vi "HART.vi"(4 "Error In":errorcluster, 7 "Command":string) -> (0 "Error Out":errorcluster, 3 "Response":string)   [LabVIEW 2018]
uses:
  MOKO_LabViewLibrary/MokoLowLevel/MokoLowLovelControl/MLLC_ConnectCluster.ctl
  MOKO_LabViewLibrary/MokoLowLevel/MokoLowLovelControl/MLLC_InterfaceType.ctl
  MOKO_LabViewLibrary/MokoLowLevel/MokoLowLovelControl/MLLC_OpenedSession.ctl
  MOKO_LabViewLibrary/MokoLowLevel/MokoLowLovelControl/MLLC_InterfaceSettings.ctl
  MOKO_LabViewLibrary/MokoLowLevel/MokoLowLovelControl/MLLC_InterfaceKind.ctl
panel:
  in  "Settings":T6={"Saved Data"=variant, "Data"={"Connect"={"InterfaceType"=enum."VISA", "OpenedSession"="", "InterfaceSettings"={"Interface"=enum."RS232", "EOS 4 read"=enum."LF (\\n)", "EOS 4 write"=enum."LF (\\n)", "TMO, ms"=10000, "Sett"=variant(cluster{"Baud Rate":u32, "Data Bits":u16, "Parity":u16, "Stop Bits":u16, "Flow Control":u16, "Eho":bool} {"Baud Rate"=75, "Data Bits"=0, "Parity"=0, "Stop Bits"=0, "Flow Control"=0, "Eho"=FALSE})}}, "Value"={"I"=0.0, "P"=0.0, "T"=0.0}, "String"="empty"}}
  in  "Error Code":u32
  in  "Driver Name":string="HART"
  in  "Mode":T7(ring)=enum."Check"
  # "HART"
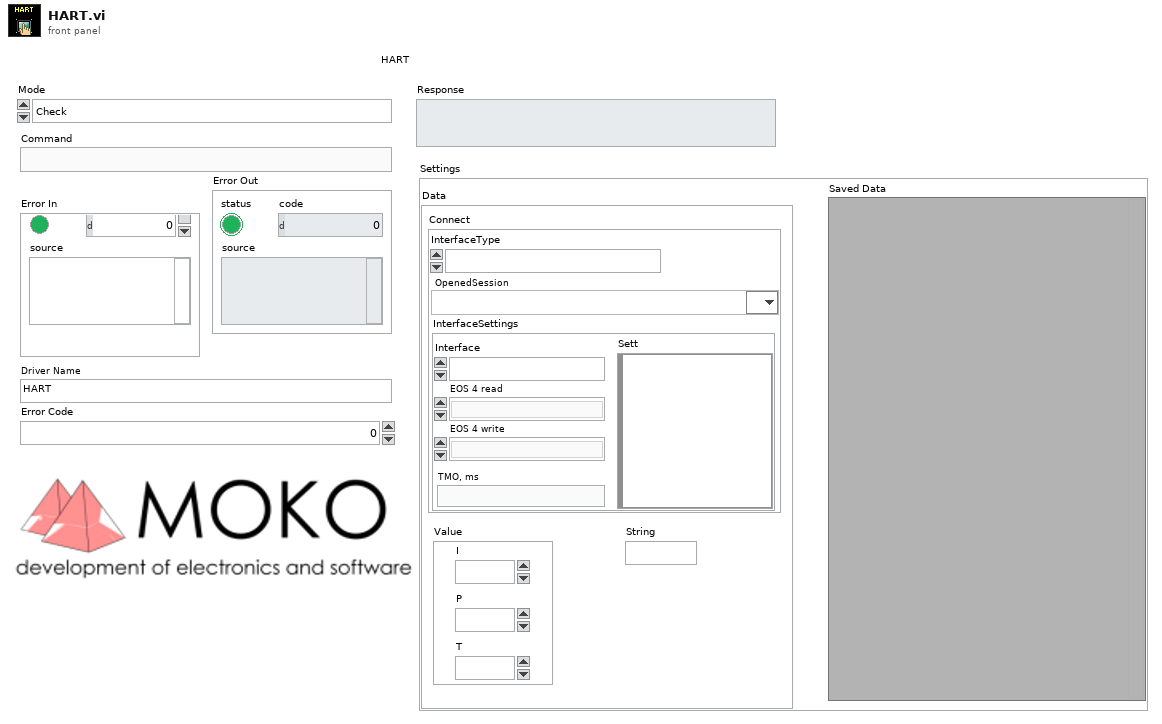
[diagram p1: front panel]
types:
  T1 = typedef "MLLC_ConnectCluster.ctl" = cluster{"InterfaceType":T2, "OpenedSession":T3, "InterfaceSettings":T4}
  T2 = typedef "MLLC_InterfaceType.ctl" = enum16{"VISA", "Prologix USB-GPIB"}
  T3 = typedef "MLLC_OpenedSession.ctl" = refnum<visa-resource-name>
  T4 = typedef "MLLC_InterfaceSettings.ctl" = cluster{"Interface":T5, "EOS 4 read":enum16{"Default (=EOS 4 write)", "CR (\\r)", "LF (\\n)", "None"}, "EOS 4 write":enum16{"CR+LF (\\r\\n)", "CR (\\r)", "LF (\\n)", "None"}, "TMO, ms":i32, "Sett":variant}
  T5 = typedef "MLLC_InterfaceKind.ctl" = enum16{"RS232", "GPIB", "USB", "Ethernet", "another"}
  T6 = cluster{"Saved Data":variant, "Data":cluster{"Connect":T1, "Value":cluster{"I":dbl, "P":dbl, "T":dbl}, "String":string}}
  T7 = enum16{"get", "set", "close", "Init", "Check", "ID"}
  T8 = cluster{"Connect":T1, "Value":cluster{"I":dbl, "P":dbl, "T":dbl}, "String":string}
  T9 = typedef "MLLC_Mode.ctl" = enum16{"get", "set", "close", "Init", "Check"}
  T10 = typedef "MLLC_Error.ctl" = errorcluster
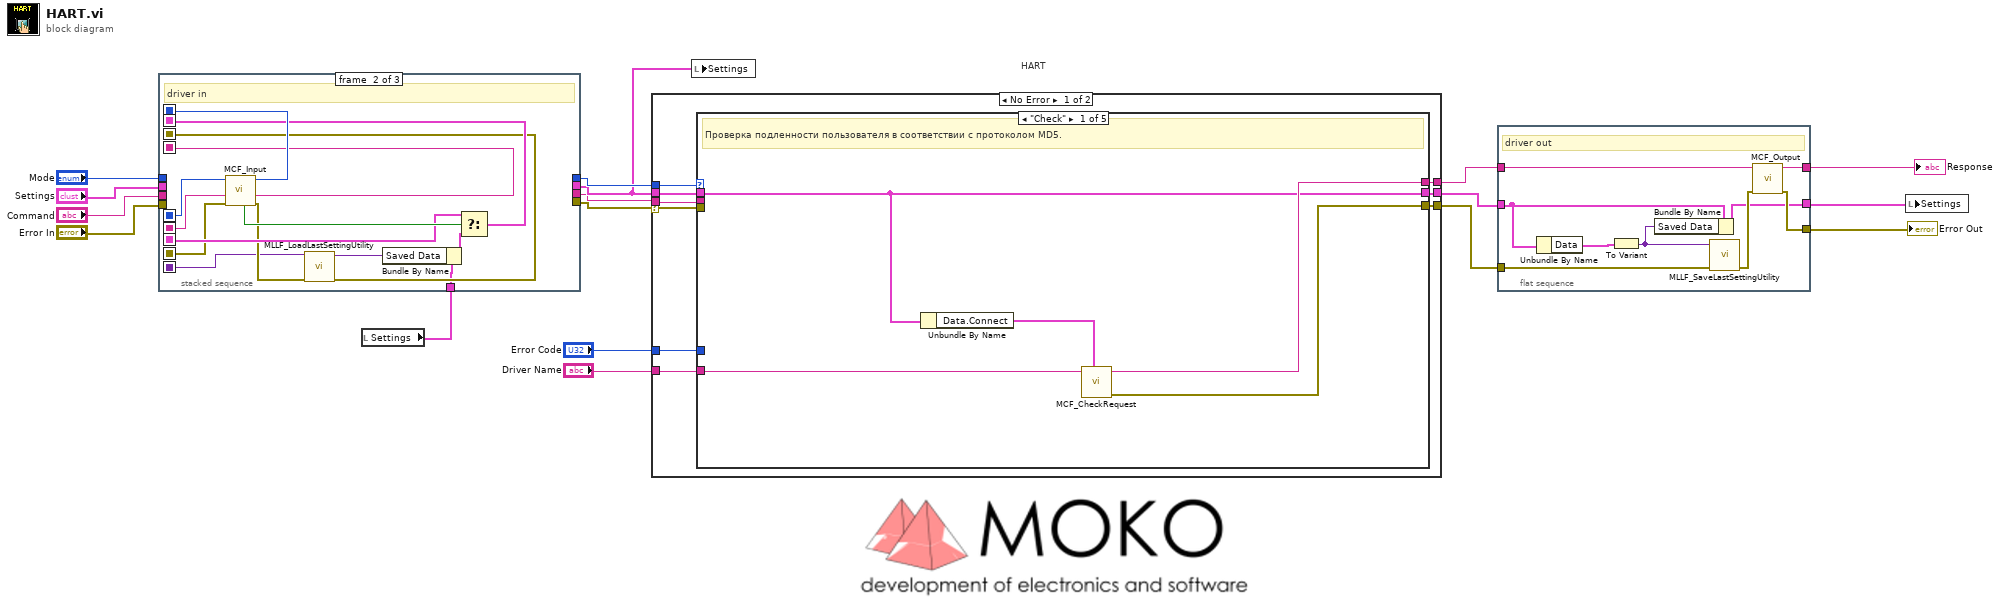
[diagram p0: block diagram]
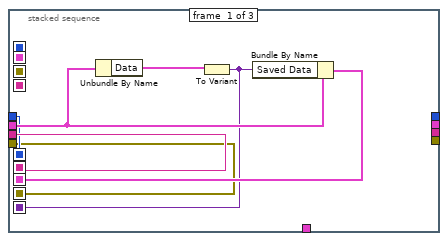
[diagram p2: hidden frame]
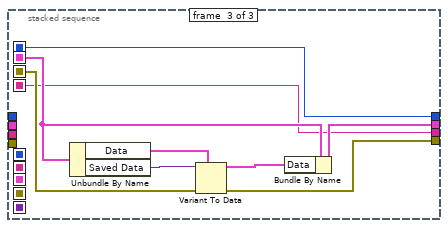
[diagram p3: hidden frame]
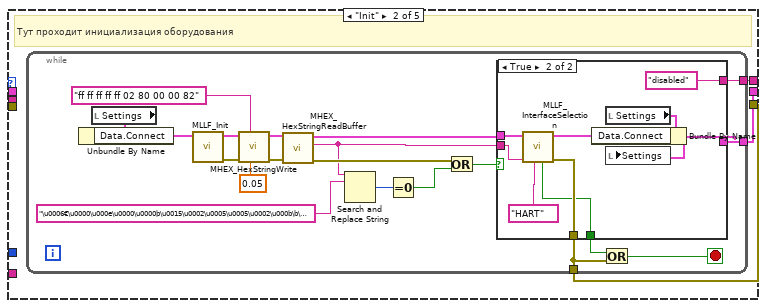
[diagram p4: hidden frame]
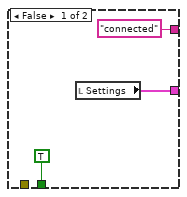
[diagram p5: hidden frame]
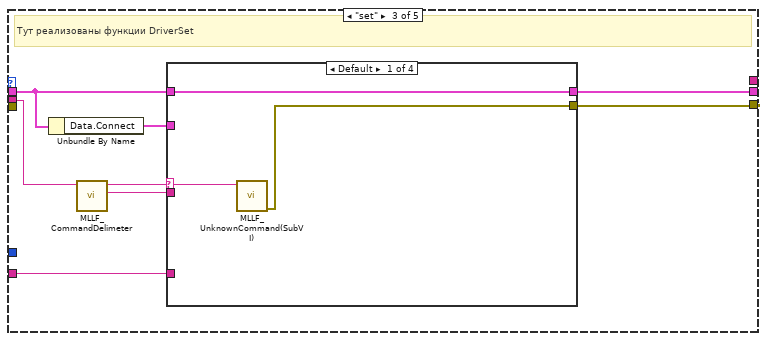
[diagram p6: hidden frame]
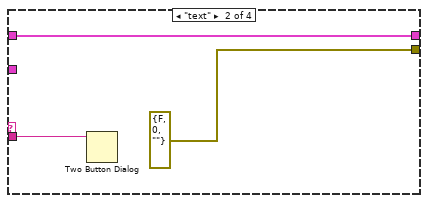
[diagram p7: hidden frame]
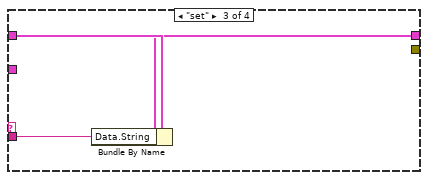
[diagram p8: hidden frame]
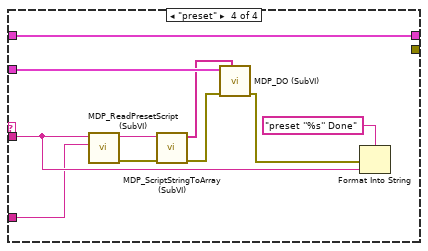
[diagram p9: hidden frame]
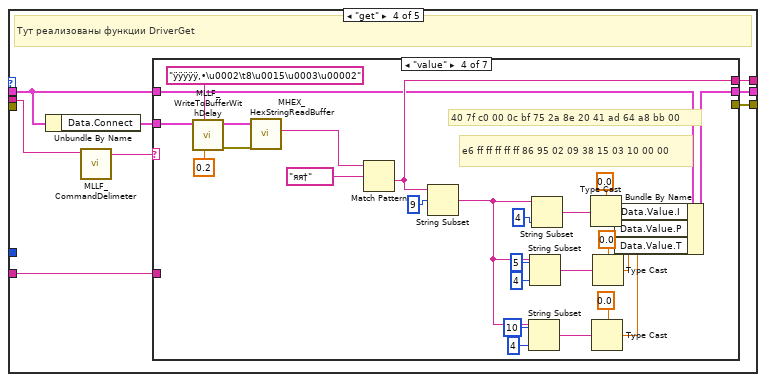
[diagram p10: hidden frame]
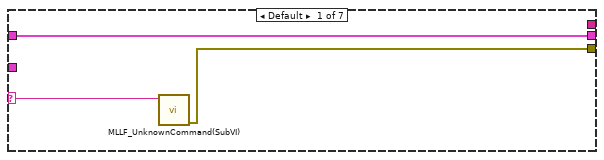
[diagram p11: hidden frame]
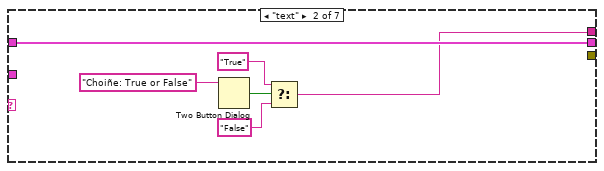
[diagram p12: hidden frame]
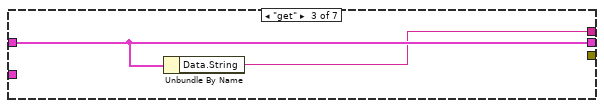
[diagram p13: hidden frame]
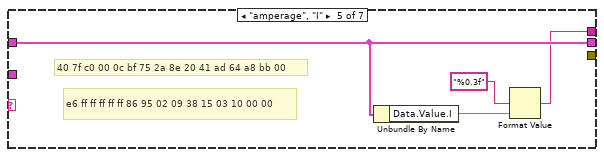
[diagram p14: hidden frame]
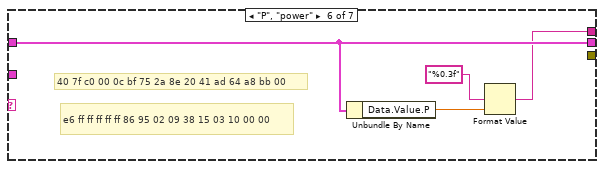
[diagram p15: hidden frame]
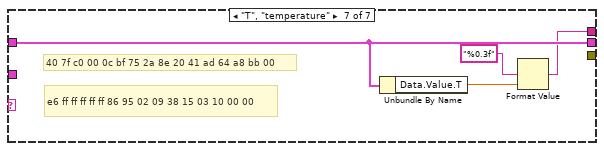
[diagram p16: hidden frame]
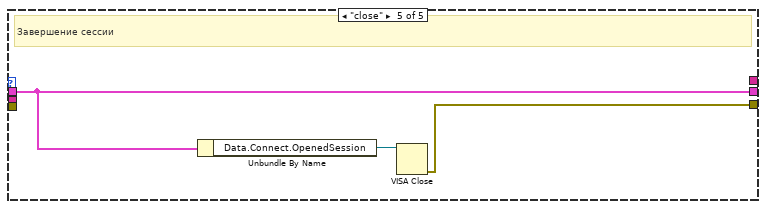
[diagram p17: hidden frame]
diagram:
  # "HART"
  n1 = local read "Settings"() -> (w13:T6)
  n2 = stacked-sequence {
    seq-local: [w20 _ _] -> [_ w36 _]
    seq-local: [w19 _ _] -> [_ w37 _]
    seq-local: [w22 _ _] -> [_ w32 _]
    seq-local: [w18 _ _] -> [_ w31 _]
    seq-local: [w21 _ _] -> [_ w27 _]
    seq-local: [_ w28 _] -> [_ _ w44]
    seq-local: [_ w38 _] -> [_ _ w41]
    seq-local: [_ w35 _] -> [_ _ w40]
    seq-local: [_ w34 _] -> [_ _ w45]
    tunnel: "Command" -> [w20 _ _]
    tunnel: "Mode" -> [w19 _ _]
    tunnel: "Error In" -> [w18 _ _]
    tunnel: "Settings" -> [w23 _ _]
    tunnel: w13 -> [_ w26 _]
    tunnel: [_ _ w40] -> w12
    tunnel: [_ _ w43] -> w14
    tunnel: [_ _ w42] -> w11
    tunnel: [_ _ w41] -> w15
    frame #0 {
      n3 = Unbundle By Name(w23) -> ("Data"=w24:T8)
      n4 = To Variant(anything=w24) -> (Variant=w21:variant)
      n5 = Bundle By Name(cluster=w23, "Saved Data"=w21) -> (w22:T6)
    }
    frame #1 {
      # "driver in"
      n6 = call "MCF_Input.vi"("Error In"=w31, "Command in"=w36, "Mode in"=w37) -> ("Error Out"=w30:errorcluster, "Command out"=w35:string, "Mode out"=w38:T9, "Boolean"=w33:bool)  [unwired: 5 in]
      n7 = call "MLLF_LoadLastSettingUtility.vi"("Error In"=w30, "Save data in"=w27) -> ("Error Out"=w28:errorcluster, "Save data out"=w25:variant)  [unwired: 8 in]
      n8 = Bundle By Name(cluster=w26, "Saved Data"=w25) -> (w29:T6)
      n9 = Select(t=w32, s=w33, f=w29) -> (s? t:f=w34:T6)
    }
    frame #2 {
      n10 = Unbundle By Name(w45) -> ("Data"=w46:T8, "Saved Data"=w39:variant)
      n11 = Variant To Data(error in=w44, type=w46, Variant=w39) -> (data=w47:T8, error out=w42:errorcluster)
      n12 = Bundle By Name(cluster=w45, "Data"=w47) -> (w43:T6)
    }
  }
  n13 = case shown="No Error" w11 {
    selector: w11 -> [w53 w185]
    tunnel: [w48 w185] -> w4
    tunnel: w15 -> [w56 _]
    tunnel: [w55 _] -> w6
    tunnel: w12 -> [w54 _]
    tunnel: w14 -> [w50 w184]
    tunnel: "Error Code" -> [w52 _]
    tunnel: "Driver Name" -> [w51 _]
    tunnel: [w49 w184] -> w5
    frame No Error {
      n14 = case shown="\"Check\"" w56 {
        tunnel: [w60 w63 _ w125 _] -> w55
        tunnel: w54 -> [_ _ w100 w128 _]
        tunnel: w53 -> [_ _ _ _ _]
        tunnel: w52 -> [_ _ _ _ _]
        tunnel: w51 -> [w61 _ w102 w126 _]
        tunnel: w50 -> [w58 _ w104 w131 w182]
        tunnel: [w58 w64 w103 w130 w182] -> w49
        tunnel: [w59 w62 w97 w124 w181] -> w48
        frame "Check" {
          # "Проверка подленности пользователя в соответствии с протоколом MD5."
          n15 = Unbundle By Name(w58) -> ("Data.Connect"=w57:T1)
          n16 = call "MCF_CheckRequest.vi"("Permanent data.Connect"=w57, "Driver Name"=w61) -> ("Error Out"=w59:errorcluster, "Output String"=w60:string)  [unwired: 8 in]
        }
        frame "Init" {
          # "Тут проходит инициализация оборудования"
          n17 = while {
            tunnel: [w81] -> w64
            tunnel: [w79] -> w63
            tunnel: [w66] -> w62
            stop <- w83 stop-if-true
            n18 = local read "Settings"() -> (w82:T6)
            n19 = Unbundle By Name(w82) -> ("Data.Connect"=w80:T1)
            n20 = call "MLLF_Init.vi"("DriverConnect in"=w80) -> ("Error Out"=w76:errorcluster, "DriverConnect out"=w77:T1)  [unwired: 7 in]
            n21 = call "MHEX_HexStringWrite.vi"("Delay Time (s)"=0.05, "Command"="ff ff ff ff ff 02 80 00 00 82" ("commands"), "error in"=w76, "DriverConnect in"=w77) -> ("error out"=w74:T10, "DriverConnect out"=w75:T1)  [unwired: 6 in]
            n22 = call "MHEX_HexStringReadBuffer.vi"("error in"=w74, "DriverConnect in"=w75) -> ("error out"=w69:T10, "String from device out"=w65:string, "DriverConnect out"=w73:T1)  [unwired: 6 in, 1 out]
            n23 = Search and Replace String(input string=w65, search string="\u0006€\u0000\u000e\u0000\u0000þ\u0015\u0002\u0005\u0005\u0002\u000b\b\u0000\t8\u0015D\u0000") -> (number of replacements=w71:i32)  [unwired: 6 in, 3 out]
            n24 = Equal To 0?(x=w71) -> (x = 0?=w70:bool)
            n25 = Or(x=w69, y=w70) -> (x .or. y?=w68:bool)
            n26 = case shown="True" w68 {
              tunnel: w73 -> [_ w95]
              tunnel: [TRUE w90] -> w84
              tunnel: [_ w96] -> w66
              tunnel: [w86 w91] -> w81
              tunnel: ["connected" "disabled"] -> w79
              tunnel: w65 -> [_ w88]
              frame False {
                n27 = local read "Settings"() -> (w86:T6)
              }
              frame True {
                n28 = call "MLLF_InterfaceSelection.vi"("Driver Name"="HART" ("String"), "Answer:"=w88, "DriverConnect in"=w95) -> ("error out"=w96:T10, "DriverConnect out"=w93:T1, "stop init?"=w90:bool)  [unwired: 4 in, 2 out]
                n29 = local read "Settings"() -> (w92:T6)
                n30 = Bundle By Name(cluster=w92, "Data.Connect"=w93) -> (w91:T6)
                n31 = local write "Settings"(w91) -> ()
              }
            }
            n32 = Or(x=w84, y=w66) -> (x .or. y?=w83:bool)
          }
        }
        frame "set" {
          # "Тут реализованы функции DriverSet"
          n33 = Unbundle By Name(w104) -> ("Data.Connect"=w101:T1)
          n34 = call "MLLF_CommandDelimeter.vi"("command with param"=w100) -> ("param 1"=w98:string, "command"=w99:string)  [unwired: 6 in, 3 out]
          n35 = case shown="Default" w99 {
            selector: w99 -> [w106 _ _ _]
            tunnel: [w107 w110 w112 w114] -> w103
            tunnel: w104 -> [w107 w110 w113 w114]
            tunnel: w101 -> [_ _ _ w118]
            tunnel: w98 -> [_ w108 w111 w117]
            tunnel: [w105 errorcluster {"status"=FALSE, "code"=0, "source"=""} ("error IO") _ _] -> w97
            tunnel: w102 -> [_ _ _ w116]
            frame Default {
              n36 = call "MLLF_UnknownCommand(SubVI).vi"("Unknown command"=w106) -> ("error out"=w105:errorcluster)  [unwired: 10 in]
            }
            frame "text" {
              n37 = Two Button Dialog(message=w108) -> ()  [unwired: 2 in, 1 out]
            }
            frame "set" {
              n38 = Bundle By Name(cluster=w113, "Data.String"=w111) -> (w112:T6)
            }
            frame "preset" {
              n39 = call "MDP_ReadPresetScript (SubVI).vi"("Driver Name"=w116, "String in"=w117) -> ("Error Out"=w121:errorcluster, "String out"=w122:string)  [unwired: 8 in]
              n40 = call "MDP_ScriptStringToArray (SubVI).vi"("Error In"=w121, "String script"=w122) -> ("Error Out"=w123:errorcluster, "Array script"=w115:string[])  [unwired: 8 in]
              n41 = call "MDP_DO (SubVI).vi"("Array script"=w115, "Error in (no error)"=w123, "DriverConnect in"=w118) -> ("Error Out"=w119:errorcluster)  [unwired: 7 in, 1 out]
              n42 = Format Into String(format string="preset ''%s'' Done" ("Befor substring"), error in=w119, w117) -> ()  [unwired: 1 in, 2 out]
            }
          }
        }
        frame "get" {
          # "Тут реализованы функции DriverGet"
          n43 = Unbundle By Name(w131) -> ("Data.Connect"=w129:T1)
          n44 = call "MLLF_CommandDelimeter.vi"("command with param"=w128) -> ("command"=w127:string)  [unwired: 6 in, 4 out]
          n45 = case shown="\"value\"" w127 {
            selector: w127 -> [w133 _ _ _ _ _ _]
            tunnel: w129 -> [_ _ _ w167 _ _ _]
            tunnel: w131 -> [w134 w140 w142 w148 w172 w176 w180]
            tunnel: [w134 w140 w142 w144 w172 w176 w180] -> w130
            tunnel: [_ w135 w141 w162 w169 w173 w177] -> w125
            tunnel: [w132 _ _ _ _ _ _] -> w124
            tunnel: w126 -> [_ _ _ _ _ _ _]
            frame Default {
              n46 = call "MLLF_UnknownCommand(SubVI).vi"("Unknown command"=w133) -> ("error out"=w132:errorcluster)  [unwired: 10 in]
            }
            frame "text" {
              n47 = Two Button Dialog(message="Choiñe: True or False") -> (T button?=w139:bool)  [unwired: 2 in]
              n48 = Select(t="True" ("string"), s=w139, f="False" ("string")) -> (s? t:f=w135:string)
            }
            frame "get" {
              n49 = Unbundle By Name(w142) -> ("Data.String"=w141:string)
            }
            frame "value" {
              # "40 7f c0 00 0c bf 75 2a 8e 20 41 ad 64 a8 bb 00"
              # "e6 ff ff ff ff ff 86 95 02 09 38 15 03 10 00 00"
              n50 = call "MLLF_WriteToBufferWithDelay.vi"("Delay Time ( 0,05 s)"=0.2 ("Delay Time (s)"), "Command"="ÿÿÿÿÿ‚•\u0002\t8\u0015\u0003\u00002", "DriverConnect in"=w167) -> ("Error Out"=w165:errorcluster, "DriverConnect out"=w166:T1)  [unwired: 7 in]
              n51 = call "MHEX_HexStringReadBuffer.vi"("error in"=w165, "DriverConnect in"=w166) -> ("String from device out"=w143:string)  [unwired: 6 in, 3 out]
              n52 = Match Pattern(string=w143, regular expression="яя†" ("HEX Response")) -> (after substring=w162:string)  [unwired: 1 in, 3 out]
              n53 = String Subset(string=w162, offset (0)=9) -> (substring=w150:string)  [unwired: 1 in]
              n54 = String Subset(string=w150, offset (0)=10, length (rest)=4 ("offset (0)")) -> (substring=w149:string)
              n55 = String Subset(string=w150, offset (0)=5, length (rest)=4 ("offset (0)")) -> (substring=w155:string)
              n56 = String Subset(string=w150, length (rest)=4 ("offset (0)")) -> (substring=w158:string)  [unwired: 1 in]
              n57 = Type Cast(type=sgl 0.0, x=w158) -> (*(type *) &x=w147:sgl)
              n58 = Type Cast(type=sgl 0.0, x=w149) -> (*(type *) &x=w145:sgl)
              n59 = Type Cast(type=sgl 0.0, x=w155) -> (*(type *) &x=w146:sgl)
              n60 = Bundle By Name(cluster=w148, "Data.Value.I"=w147, "Data.Value.P"=w146, "Data.Value.T"=w145) -> (w144:T6)
            }
            frame "amperage", "I" {
              # "40 7f c0 00 0c bf 75 2a 8e 20 41 ad 64 a8 bb 00"
              # "e6 ff ff ff ff ff 86 95 02 09 38 15 03 10 00 00"
              n61 = Unbundle By Name(w172) -> ("Data.Value.I"=w171:dbl)
              n62 = Format Value(format string="%0.3f", value (0)=w171) -> (output string=w169:string)  [unwired: 1 in]
            }
            frame "P", "power" {
              # "40 7f c0 00 0c bf 75 2a 8e 20 41 ad 64 a8 bb 00"
              # "e6 ff ff ff ff ff 86 95 02 09 38 15 03 10 00 00"
              n63 = Unbundle By Name(w176) -> ("Data.Value.P"=w175:dbl)
              n64 = Format Value(format string="%0.3f", value (0)=w175) -> (output string=w173:string)  [unwired: 1 in]
            }
            frame "T", "temperature" {
              # "40 7f c0 00 0c bf 75 2a 8e 20 41 ad 64 a8 bb 00"
              # "e6 ff ff ff ff ff 86 95 02 09 38 15 03 10 00 00"
              n65 = Unbundle By Name(w180) -> ("Data.Value.T"=w179:dbl)
              n66 = Format Value(format string="%0.3f", value (0)=w179) -> (output string=w177:string)  [unwired: 1 in]
            }
          }
        }
        frame "close" {
          # "Завершение сессии"
          n67 = Unbundle By Name(w182) -> ("Data.Connect.OpenedSession"=w183:T3)
          n68 = VISA Close(VISA resource name=w183) -> (error out=w181:errorcluster)  [unwired: 1 in]
        }
      }
    }
    frame Error {
    }
  }
  n69 = local write "Settings"(w14) -> ()
  n70 = flat-sequence {
    tunnel: [w194] -> w3
    tunnel: [w193] -> w1
    tunnel: w6 -> [w192]
    tunnel: w4 -> [w191]
    tunnel: w5 -> [w187]
    tunnel: [w189] -> w2
    frame #0 {
      # "driver out"
      n71 = Unbundle By Name(w187) -> ("Data"=w186:T8)
      n72 = To Variant(anything=w186) -> (Variant=w188:variant)
      n73 = Bundle By Name(cluster=w187, "Saved Data"=w188) -> (w189:T6)
      n74 = call "MLLF_SaveLastSettingUtility.vi"("error in"=w191, "Saved Data"=w188) -> ("error out"=w190:T10)  [unwired: 8 in, 1 out]
      n75 = call "MCF_Output.vi"("Error In"=w190, "Input"=w192) -> ("Error Out"=w193:errorcluster, "Output"=w194:string)  [unwired: 8 in]
    }
  }
  n76 = local write "Settings"(w2) -> ()
  "Response" <- w3
  "Error Out" <- w1
